vi "dfd_FXP Direct IIR I with IS.vi"(6 "state in":i64[](array[numeric]), 7 "FXPOPs":T1[](array[typedef]) {"source" items=["Coef a/k"=0, "Coef b/v"=7, "Input"=1, "Output"=2, "Multiplicand"=3, "Product"=4, "Sum"=5, "Delay"=6, "Gain"=8]}, 8 "filtering statistics in":T6(array[cluster]) {"statistics information"."min value" format="%.2f"; "statistics information"."max value" format="%.2f"; "Quantizer Source" items=["Coefficients a/k"=0, "Coefficients b/v"=7, "Input"=1, "Output"=2, "Multiplicand"=3, "Product"=4, "Sum"=5, "Delay"=6]}, 9 "coef a":T7, 10 "coef b":T7, 11 "X":T7) -> (0 "filtering statistics out":T6(array[cluster]) {"statistics information"."min value" format="%.2f"; "statistics information"."max value" format="%.2f"; "Quantizer Source" items=["Coefficients a/k"=0, "Coefficients b/v"=7, "Input"=1, "Output"=2, "Multiplicand"=3, "Product"=4, "Sum"=5, "Delay"=6]}, 3 "filtered X":T7, 4 "state out":i64[](array[numeric]))   [LabVIEW 2017, in "NI_DigFilter_FXP.lvlib"]
uses:
  <vilib>/addons/Digital Filter Design/NI_DigFilter_FXP.lvlib
  <vilib>/addons/Digital Filter Design/_Objects.llb/dfd_DFXP Data Type (vector).ctl
  <vilib>/addons/Digital Filter Design/_Objects.llb/DFD Quantization Sources.ctl
  <vilib>/addons/Digital Filter Design/_Objects.llb/DFD FXP Statistics Data.ctl
  <vilib>/addons/Digital Filter Design/_Objects.llb/dfd_DFXP Data Type (scaler).ctl
  <vilib>/addons/Digital Filter Design/_Objects.llb/dfd_DFXP Operation Parameter.ctl
  <vilib>/addons/Digital Filter Design/_Objects.llb/dfd_Internal Quantization Srcs.ctl
  <vilib>/addons/Digital Filter Design/NI_DigFilterLicensed.lvlib
panel:
  in  "DFXP Value":T3={"value"=0, "wl"=0, "iwl"=0, "Signed"=TRUE} {"value" format="%.0x"}
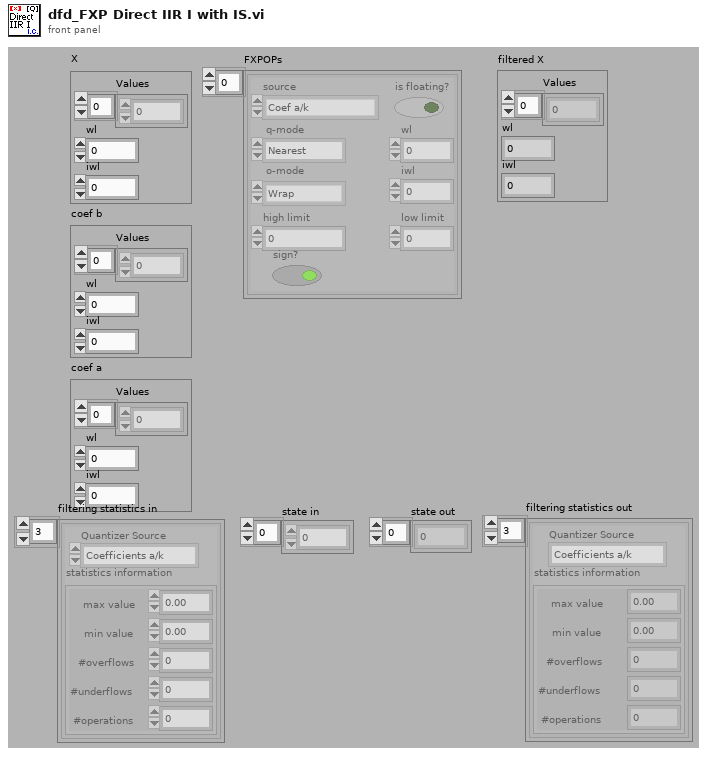
[diagram p1: front panel]
types:
  T1 = typedef "dfd_DFXP Operation Parameter.ctl" = cluster{"source":T2, "is floating?":bool, "o-mode":enum16{"Saturation", "Wrap"}, "q-mode":enum16{"Nearest", "Truncation"}, "wl":i16, "high limit":i64, "low limit":i64, "iwl":i16, "sign?":bool}
  T2 = typedef "NI_DigFilterLicensed.lvlib/dfd_Internal Quantization Srcs.ctl" = u16
  T3 = typedef "dfd_DFXP Data Type (scaler).ctl" = cluster{"value":i64, "wl":i16, "iwl":i16, "Signed":bool}
  T4 = typedef "NI_DigFilterLicensed.lvlib/DFD Quantization Sources.ctl" = u16
  T5 = typedef "NI_DigFilterLicensed.lvlib/DFD FXP Statistics Data.ctl" = cluster{"max value":ext, "min value":ext, "#overflows":i32, "#underflows":i32, "#operations":i32}
  T6 = cluster{"Quantizer Source":T4, "statistics information":T5}[]
  T7 = typedef "dfd_DFXP Data Type (vector).ctl" = cluster{"Values":i64[], "wl":i16, "iwl":i16}
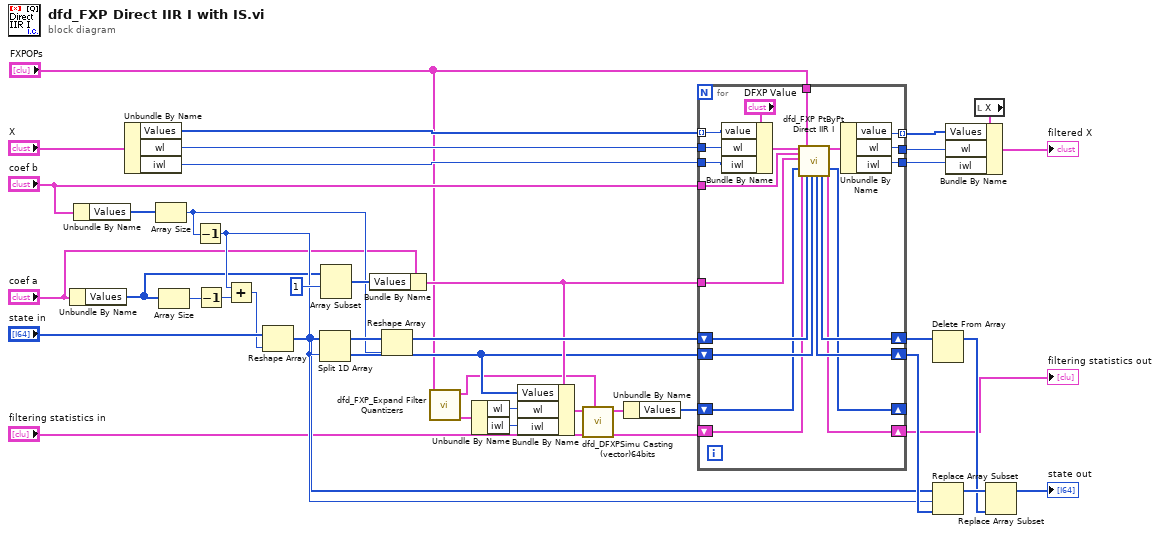
[diagram p0: block diagram]
diagram:
  n1 = Unbundle By Name("coef a") -> ("Values"=w21:i64[])
  n2 = Unbundle By Name("coef b") -> ("Values"=w22:i64[])
  n3 = Unbundle By Name("X") -> ("Values"=w19:i64[], "wl"=w18:i16, "iwl"=w17:i16)
  n4 = Array Size(array=w22) -> (size(s)=w25:i32)
  n5 = Array Size(array=w21) -> (size(s)=w41:i32)
  n6 = Decrement(x=w25) -> (x-1=w28:i32)
  n7 = Decrement(x=w41) -> (x-1=w39:i32)
  n8 = Add(x=w28, y=w39) -> (x+y=w29:i32)
  n9 = Reshape Array("state in", w29) -> (w24:i64[])
  n10 = Split 1D Array(array=w24, index=w28) -> (first subarray=w27:i64[], second subarray=w8:i64[])
  n11 = Array Subset(array=w21, index=1) -> (w37:i64[])  [unwired: 1 in]
  n12 = Bundle By Name(cluster="coef a", "Values"=w37) -> (w12:T7)
  n13 = Reshape Array(w27, w25) -> (w26:i64[])
  n14 = call <vilib>:"dfd_FXP_Expand Filter Quantizers.vi"("FXPOPs"="FXPOPs") -> ("Delay"=w11:T1, "Multiplicand"=w4:T1)  [unwired: 9 out]
  n15 = Unbundle By Name(w11) -> ("wl"=w10:i16, "iwl"=w9:i16)
  n16 = Bundle By Name(cluster=w12, "Values"=w8, "wl"=w10, "iwl"=w9) -> (w7:T7)
  n17 = call <vilib>:"dfd_DFXPSimu Casting (vector)64bits.vi"("op params"=w4, "filtering statistics in"="filtering statistics in", "Value in"=w7) -> ("filtering statistics out"=w5:T6, "Value out"=w3:T7)  [unwired: 1 in, 6 out]
  n18 = Unbundle By Name(w3) -> ("Values"=w2:i64[])
  n19 = for {
    tunnel: w19 -> [w62] mode=indexing
    tunnel: "coef b" -> [w61]
    shift-right: [w56] -> w33
    shift-left: w26 -> [w59]
    shift-right: [w57] -> w34
    shift-left: w8 -> [w58]
    tunnel: w12 -> [w60]
    tunnel: [w47] -> w35 mode=indexing
    tunnel: "FXPOPs" -> [w54]
    shift-right: [w52] -> w23
    shift-left: w5 -> [w53]
    tunnel: w18 -> [w49]
    tunnel: w17 -> [w48]
    tunnel: [w46] -> w14
    tunnel: [w45] -> w13
    shift-right: [w43] -> _
    shift-left: w2 -> [w44]
    n20 = Bundle By Name(cluster="DFXP Value", "value"=w62, "wl"=w49, "iwl"=w48) -> (w51:T3)
    n21 = call <vilib>:"dfd_FXP PtByPt Direct IIR I.vi"("x"=w51, "coef b[0..M]"=w61, "coef a[1..N]"=w60, "yState tmp in"=w44, "filtering statistics in"=w53, "FXPOPs"=w54, "xState in"=w59, "yState in"=w58) -> ("yState out"=w57:i64[], "xState out"=w56:i64[], "filtered x"=w55:T3, "yState tmp out"=w43:i64[], "filtering statistics out"=w52:T6)  [unwired: 7 out]
    n22 = Unbundle By Name(w55) -> ("value"=w47:i64, "wl"=w46:i16, "iwl"=w45:i16)
  }
  "filtering statistics out" <- w23
  n23 = Delete From Array(array=w33) -> (array with subset deleted=w31:i64[])  [unwired: 2 in, 1 out]
  n24 = Replace Array Subset(array=w24, new element=w34, index=w28) -> (w32:i64[])
  n25 = local read "X"() -> (w15:T7)
  n26 = Bundle By Name(cluster=w15, "Values"=w35, "wl"=w14, "iwl"=w13) -> (→"filtered X":T7)
  n27 = Replace Array Subset(array=w32, new element=w31) -> (→"state out":i64[])  [unwired: 1 in]
